vi "Main_12a.vi"() -> ()   [LabVIEW 2020]
uses:
  Cluster Point.ctl
  1754cb09-e69e-4dd3-b093-f66bff0fb40e.vi
  <vilib>/Comparison/Less/Less Functor/Less Functor.lvclass
panel:
  out "Array 2":i32[][](array[numeric])
  out "Map":map{T1, i32}(c390)
  out "Array":u8[][](array[numeric])
  out "End":T1
  out "Start":T1
  out "Answer":i32
  in  "Puzzle":string="abcccccccccccccccccccccccccccccccaaaaaaaaaaaaaaaaccaaaaaaaaccccccccccccccccccccccccccccccccccccaaaaaa\nabcccccccccccccccccccccccccccccccaaaaaaaaaaaaaaaaaccaaaaaaccccccccccccccccccccccccccccccccccccccaaaaa\nabcccccccccccccccccccccccccccccccccaaaaaaaacccaaaaccaaaaaaccccccccccccccccccccaaaccccccccccccccccaaaa\nabcccccccccccccccccccccccccccccccccccaaaaaaaccaaccccaaaaaaccccccccccccccccccccaaaccccccccccccccccaaaa\nabcccccccccccccccccccccccccccccaaacccaaaaaaaacccccccaaccaaccccccccccccccccccccaaaccccccccccccccccaaac\nabcccccccccccccccccccccccccccccaaaaaaaaacaaaacccccccccccccccaccaaccccccccccccciiaaccaaaccc..."
  in  "Example":string="Sabqponm\nabcryxxl\naccszExk\nacctuvwj\nabdefghi"
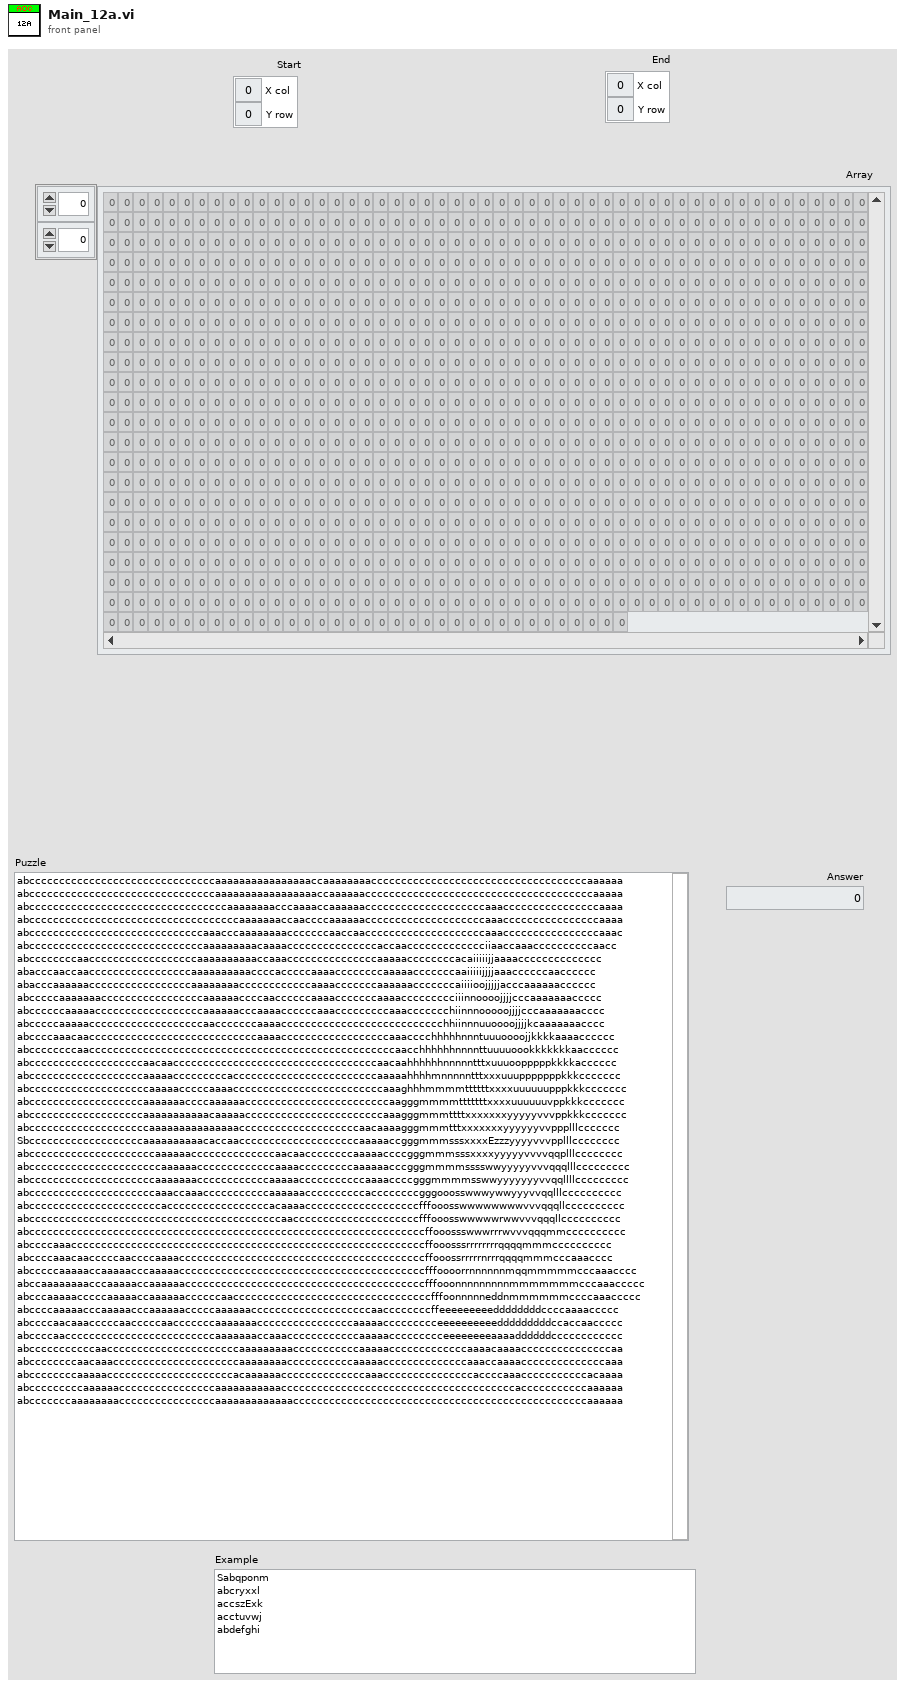
[diagram p1: front panel]
types:
  T1 = typedef "Cluster Point.ctl" = cluster{"X col":i32, "Y row":i32}
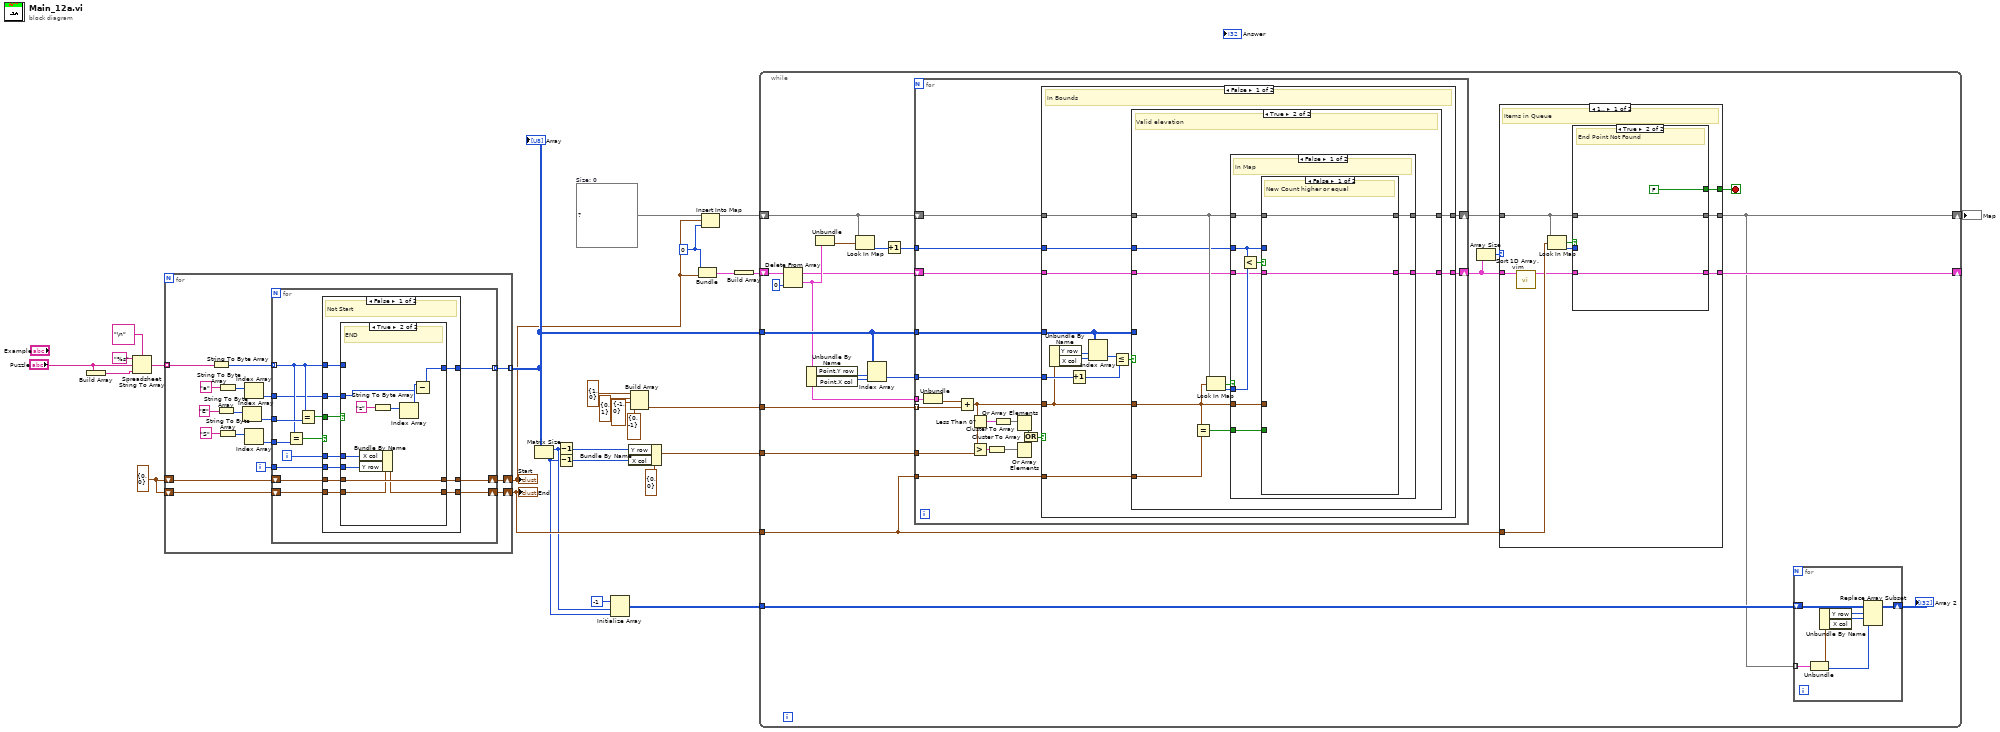
[diagram p0: block diagram]
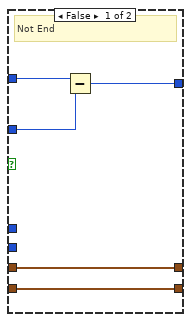
[diagram p2: hidden frame]
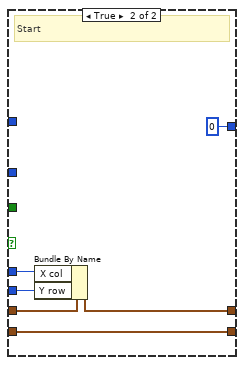
[diagram p3: hidden frame]
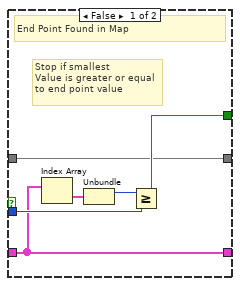
[diagram p4: hidden frame]
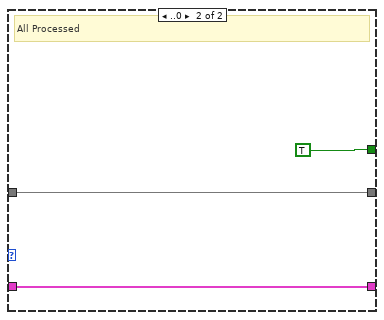
[diagram p5: hidden frame]
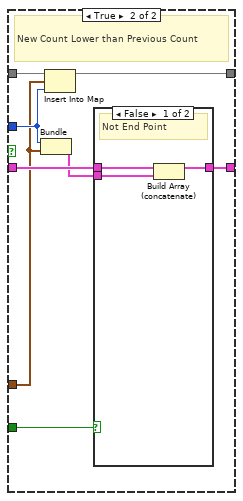
[diagram p7: hidden frame]
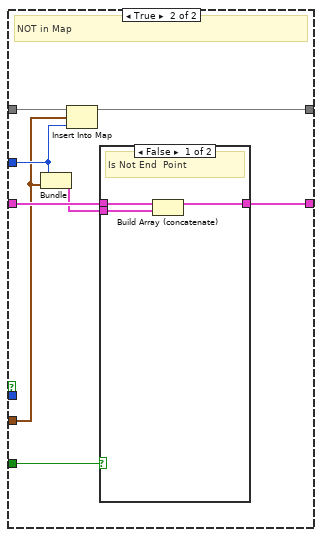
[diagram p9: hidden frame]
diagram:
  w9 = 0 ("value")
  w20 = T1 {"X col"=0, "Y row"=0} ("Point")
  w12 = map{T1, i32} {}  # Size: 0
  n1 = Build Array("Puzzle") -> (w28:string[])
  n2 = Spreadsheet String To Array(delimiter (Tab)="\n", format string="%s", spreadsheet string="Puzzle", array type (2D Dbl)=w28) -> (array=w25:string[])
  n3 = for {
    tunnel: w25 -> [w45] mode=indexing
    shift-right: [w30] -> w8
    shift-left: w20 -> [w34]
    shift-right: [w29] -> w22
    shift-left: w20 -> [w33]
    tunnel: [w31] -> w21 mode=indexing
    i -> [w32]
    n4 = String To Byte Array(string=w45) -> (unsigned byte array=w42:u8[])
    n5 = String To Byte Array(string="E") -> (unsigned byte array=w40:u8[])
    n6 = String To Byte Array(string="a") -> (unsigned byte array=w43:u8[])
    n7 = String To Byte Array(string="S") -> (unsigned byte array=w37:u8[])
    n8 = Index Array(array=w40) -> (element=w36:u8)  [unwired: 1 in]
    n9 = Index Array(array=w43) -> (element=w41:u8)  [unwired: 1 in]
    n10 = Index Array(array=w37) -> (element=w35:u8)  [unwired: 1 in]
    n11 = for {
      tunnel: w42 -> [w56] mode=indexing
      tunnel: w41 -> [w46]
      tunnel: w36 -> [w58]
      tunnel: w35 -> [w57]
      shift-right: [w51] -> w30
      shift-left: w34 -> [w50]
      shift-right: [w48] -> w29
      shift-left: w33 -> [w49]
      tunnel: w32 -> [w52]
      tunnel: [w47] -> w31 mode=indexing
      i -> [w53]
      n12 = Equal?(x=w56, y=w57) -> (x = y?=w55:bool)
      n13 = Equal?(x=w56, y=w58) -> (x = y?=w54:bool)
      n14 = case shown="False" w55 {
        tunnel: w56 -> [w67 _]
        tunnel: w54 -> [w68 _]
        tunnel: w53 -> [w65 w86]
        tunnel: w52 -> [w64 w85]
        tunnel: [w60 w87] -> w51
        tunnel: w50 -> [w62 w88]
        tunnel: w49 -> [w61 w89]
        tunnel: [w63 w89] -> w48
        tunnel: [w66 u8 0] -> w47
        tunnel: w46 -> [w59 _]
        frame False {
          # "Not Start"
          n15 = case shown="True" w68 {
            tunnel: w67 -> [w73 _]
            tunnel: [w71 w74] -> w66
            tunnel: w65 -> [_ w77]
            tunnel: w64 -> [_ w78]
            tunnel: [w69 w80] -> w63
            tunnel: w62 -> [w70 w81]
            tunnel: w61 -> [w69 w79]
            tunnel: [w70 w81] -> w60
            tunnel: w59 -> [w72 w75]
            frame False {
              # "Not End"
              n16 = Subtract(x=w73, y=w72) -> (x-y=w71:u8)
            }
            frame True {
              # "END"
              n17 = Bundle By Name(cluster=w79, "X col"=w77, "Y row"=w78) -> (w80:T1)
              n18 = String To Byte Array(string="z") -> (unsigned byte array=w82:u8[])
              n19 = Index Array(array=w82) -> (element=w76:u8)  [unwired: 1 in]
              n20 = Subtract(x=w76, y=w75) -> (x-y=w74:u8)
            }
          }
        }
        frame True {
          # "Start"
          n21 = Bundle By Name(cluster=w88, "X col"=w86, "Y row"=w85) -> (w87:T1)
        }
      }
    }
  }
  "Start" <- w8
  "End" <- w22
  "Array" <- w21
  n22 = Matrix Size(0:w21) -> (1:w4:i32, 2:w3:i32)
  n23 = Decrement(x=w4) -> (x-1=w14:i32)
  n24 = Decrement(x=w3) -> (x-1=w13:i32)
  n25 = Initialize Array(-1, w4, w3) -> (w2:i32[][])
  n26 = Bundle By Name(cluster=T1 {"X col"=0, "Y row"=0} ("unsigned byte array"), "Y row"=w14, "X col"=w13) -> (w15:T1)
  n27 = Build Array(T1 {"X col"=1, "Y row"=0} ("unsigned byte array"), T1 {"X col"=0, "Y row"=1} ("unsigned byte array"), T1 {"X col"=-1, "Y row"=0} ("unsigned byte array"), T1 {"X col"=0, "Y row"=-1} ("unsigned byte array")) -> (w23:T1[])
  n28 = Bundle("value"=w9, "Point"=w8) -> (w7:cluster{"value":i32, "Point":T1})  [unwired: 1 in]
  n29 = Insert Into Map(map in=w12, key=w8, value=w9) -> (map out=w11:map{T1, i32})  [unwired: 2 out]
  n30 = Build Array(w7) -> (w10:cluster{"value":i32, "Point":T1}[])
  n31 = while {
    tunnel: w23 -> [w112]
    tunnel: w21 -> [w106]
    tunnel: w15 -> [w111]
    tunnel: w22 -> [w95]
    shift-right: [w91] -> w6
    shift-left: w11 -> [w93]
    shift-right: [w99] -> _
    shift-left: w10 -> [w104]
    tunnel: w2 -> [w92]
    stop <- w97 stop-if-true
    n32 = Delete From Array(array=w104, index=0) -> (deleted portion=w103:cluster{"value":i32, "Point":T1}, array with subset deleted=w102:cluster{"value":i32, "Point":T1}[])  [unwired: 1 in]
    n33 = Unbundle By Name(w103) -> ("Point.Y row"=w108:i32, "Point.X col"=w107:i32)
    n34 = Unbundle(w103) -> ("Point"=w96:T1)  [unwired: 1 out]
    n35 = Look In Map(map=w93, key=w96) -> (value=w110:i32)  [unwired: 1 in, 1 out]
    n36 = Index Array(array=w106, index (row)=w108, index (col)=w107) -> (element=w105:u8)
    n37 = Increment(x=w110) -> (x+1=w109:i32)
    n38 = for {
      tunnel: w112 -> [w160] mode=indexing
      tunnel: w111 -> [w143]
      tunnel: w106 -> [w151]
      tunnel: w103 -> [w156]
      shift-right: [w145] -> w98
      shift-left: w93 -> [w147]
      tunnel: w109 -> [w148]
      tunnel: w105 -> [w149]
      shift-right: [w144] -> w100
      shift-left: w102 -> [w146]
      tunnel: w95 -> [w141]
      n39 = Unbundle(w156) -> ("Point"=w142:T1)  [unwired: 1 out]
      n40 = Add(x=w142, y=w160) -> (x+y=w150:T1)
      n41 = Less Than 0?(x=w150) -> (x < 0?=w155:cluster{"X col":bool, "Y row":bool})
      n42 = Greater?(x=w150, y=w143) -> (0:w153:cluster{"X col":bool, "Y row":bool})
      n43 = Cluster To Array(cluster=w153) -> (array=w152:bool[])
      n44 = Cluster To Array(cluster=w155) -> (array=w154:bool[])
      n45 = Or Array Elements(Boolean array=w154) -> (logical OR=w158:bool)
      n46 = Or Array Elements(Boolean array=w152) -> (logical OR=w159:bool)
      n47 = Or(x=w158, y=w159) -> (x .or. y?=w157:bool)
      n48 = case shown="False" w157 {
        tunnel: w151 -> [w168 _]
        tunnel: w150 -> [w166 _]
        tunnel: w149 -> [w172 _]
        tunnel: w148 -> [w167 _]
        tunnel: w147 -> [w165 w223]
        tunnel: w146 -> [w164 w222]
        tunnel: [w163 w223] -> w145
        tunnel: [w162 w222] -> w144
        tunnel: w141 -> [w161 _]
        frame False {
          # "In Bounds"
          n49 = Unbundle By Name(w166) -> ("Y row"=w173:i32, "X col"=w174:i32)
          n50 = Increment(x=w172) -> (x+1=w170:u8)
          n51 = Index Array(array=w168, index (row)=w173, index (col)=w174) -> (element=w171:u8)
          n52 = Less Or Equal?(x=w171, y=w170) -> (x <= y?=w169:bool)
          n53 = case shown="True" w169 {
            tunnel: w168 -> [_ _]
            tunnel: w167 -> [_ w185]
            tunnel: w166 -> [_ w178]
            tunnel: w165 -> [w176 w186]
            tunnel: w164 -> [w175 w184]
            tunnel: [w176 w183] -> w163
            tunnel: [w175 w182] -> w162
            tunnel: w161 -> [_ w179]
            frame False {
              # "Point too High"
            }
            frame True {
              # "Valid elevation"
              n54 = Equal?(x=w178, y=w179) -> (x = y?=w177:bool)
              n55 = Look In Map(map=w186, key=w178) -> (key not found?=w181:bool, value=w180:i32)  [unwired: 1 in]
              n56 = case shown="False" w181 {
                tunnel: w180 -> [w195 _]
                tunnel: w186 -> [w193 w217]
                tunnel: w178 -> [w189 w212]
                tunnel: w185 -> [w190 w213]
                tunnel: w184 -> [w191 w215]
                tunnel: [w192 w216] -> w183
                tunnel: [w188 w214] -> w182
                tunnel: w177 -> [w187 w210]
                frame False {
                  # "In Map"
                  n57 = Less?(x=w190, y=w195) -> (x < y?=w194:bool)
                  n58 = case shown="False" w194 {
                    tunnel: w193 -> [w197 w205]
                    tunnel: [w197 w204] -> w192
                    tunnel: w191 -> [w196 w203]
                    tunnel: w190 -> [_ w201]
                    tunnel: w189 -> [_ w199]
                    tunnel: [w196 w202] -> w188
                    tunnel: w187 -> [_ w198]
                    frame False {
                      # "New Count higher or equal"
                    }
                    frame True {
                      # "New Count Lower than Previous Count"
                      n59 = Bundle(w201, "Point"=w199) -> (w200:cluster{i32, "Point":T1})  [unwired: 1 in]
                      n60 = Insert Into Map(map in=w205, key=w199, value=w201) -> (map out=w204:map{T1, i32})  [unwired: 2 out]
                      n61 = case shown="False" w198 {
                        tunnel: w203 -> [w208 w209]
                        tunnel: [w207 w209] -> w202
                        tunnel: w200 -> [w206 _]
                        frame False {
                          # "Not End Point"
                          n62 = Build Array (concatenate)(w208, w206) -> (w207:cluster{"value":i32, "Point":T1}[])
                        }
                        frame True {
                          # "Is End Point"
                        }
                      }
                    }
                  }
                }
                frame True {
                  # "NOT in Map"
                  n63 = Bundle(w213, "Point"=w212) -> (w211:cluster{i32, "Point":T1})  [unwired: 1 in]
                  n64 = Insert Into Map(map in=w217, key=w212, value=w213) -> (map out=w216:map{T1, i32})  [unwired: 2 out]
                  n65 = case shown="False" w210 {
                    tunnel: w215 -> [w220 w221]
                    tunnel: [w219 w221] -> w214
                    tunnel: w211 -> [w218 _]
                    frame False {
                      # "Is Not End  Point"
                      n66 = Build Array (concatenate)(w220, w218) -> (w219:cluster{"value":i32, "Point":T1}[])
                    }
                    frame True {
                      # "Is End Point"
                    }
                  }
                }
              }
            }
          }
        }
        frame True {
          # "Out Of Bounds"
        }
      }
    }
    n67 = Array Size(array=w100) -> (size(s)=w101:i32)
    n68 = case shown="1.." w101 {
      tunnel: w100 -> [w120 w140]
      tunnel: [w122 w140] -> w99
      tunnel: w98 -> [w126 w139]
      tunnel: [w124 w139] -> w91
      tunnel: [w123 TRUE] -> w97
      tunnel: w95 -> [w128 _]
      frame 1.. {
        # "Items in Queue"
        n69 = call "Sort 1D Array.vim"("unsorted array"=w120) -> ("sorted array"=w121:cluster{"value":i32, "Point":T1}[])  [unwired: 10 in]
        n70 = Look In Map(map=w126, key=w128) -> (key not found?=w127:bool, value=w125:i32)  [unwired: 1 in]
        n71 = case shown="True" w127 {
          tunnel: w126 -> [w130 w137]
          tunnel: w125 -> [w132 _]
          tunnel: [w130 w137] -> w124
          tunnel: [w131 FALSE] -> w123
          tunnel: w121 -> [w129 w135]
          tunnel: [w129 w135] -> w122
          frame False {
            # "Stop if smallest\nValue is greater or equal\nto end point value"
            # "End Point Found in Map"
            n72 = Index Array(array=w129) -> (element=w134:cluster{"value":i32, "Point":T1})  [unwired: 1 in]
            n73 = Unbundle(w134) -> ("value"=w133:i32)  [unwired: 1 out]
            n74 = Greater Or Equal?(x=w133, y=w132) -> (x >= y?=w131:bool)
          }
          frame True {
            # "End Point Not Found"
          }
        }
      }
      frame ..0 {
        # "All Processed"
      }
    }
    n75 = for {
      tunnel: w91 -> [w119] mode=indexing
      shift-right: [w117] -> w90
      shift-left: w92 -> [w118]
      n76 = Unbundle(w119) -> ("Point"=w116:T1, "min step"=w113:i32)
      n77 = Unbundle By Name(w116) -> ("Y row"=w115:i32, "X col"=w114:i32)
      n78 = Replace Array Subset(array=w118, new element=w113, index (row)=w115, index (col)=w114) -> (w117:i32[][])
    }
    "Array 2" <- w90
  }
  "Map" <- w6
